vi "Process.vi"(8 "error in":errorcluster, 11 "SMO.SelfTerminating":refnum<class "SMO.SelfTerminating.lvclass">) -> (0 "error out":errorcluster, 3 "SMO.SelfTerminating out":refnum<class "SMO.SelfTerminating.lvclass">)   [LabVIEW 2013, in "SMO.SelfTerminating.lvclass"]
uses:
  SMO.SelfTerminating.lvclass
  SMO/Typedefs/Parent Call--Enum.ctl
  SMO/SMO.lvclass
panel:
  # "For instructions on how to use the JKI State Machine Objects, examples and video tutorials, visit:\nhttp://jki.net/state-machine-objects/\n\nJKI State Machine Objects™\nhttp://jki.net/state-machine-objects/\nCopyright (C) 2005-2015, JKI <info@jki.net>\nALL RIGHTS RESERVED"
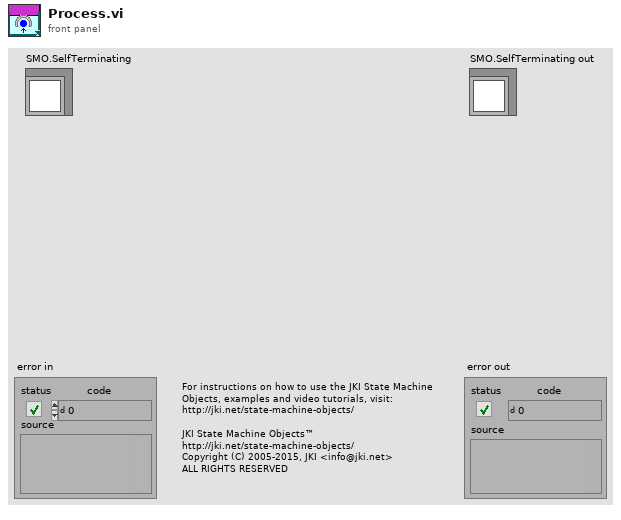
[diagram p1: front panel]
types:
  T1 = typedef "SMO.lvclass/Parent Call--Enum.ctl" = enum16{"Allows parent to run", "Does not request parent to run"}
  T2 = typedef "SMO.lvclass/Protected Events.ctl" = cluster{"StopProcesses":refnum<user-event>, "AbortProcesses":refnum<user-event>, "Config Changed":refnum<user-event>, "Dependency":refnum<user-event>}
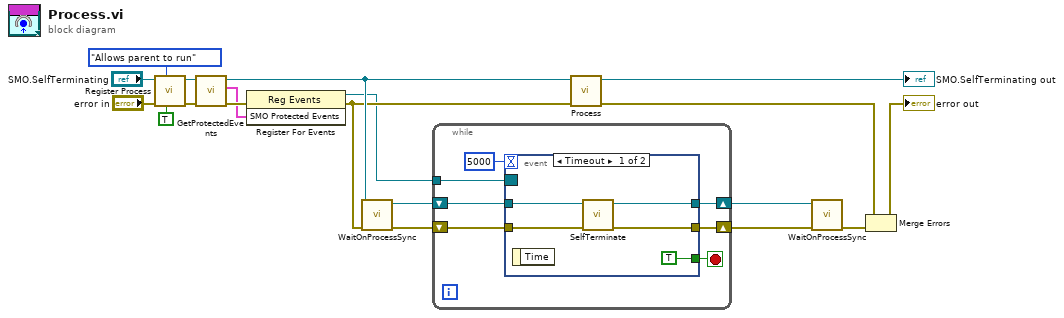
[diagram p0: block diagram]
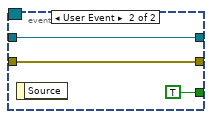
[diagram p2: hidden frame]
diagram:
  n1 = call "Register Process.vi"("Forces Self to Run (F)"=TRUE, "Parent Call"=Parent_Call--Enum."Allows parent to run", "error in (no error)"="error in", "SMO"="SMO.SelfTerminating") -> ("error out"=w9:errorcluster, "SMO out"=w11:refnum<class "SMO.SelfTerminating.lvclass">)  [unwired: 6 in]
  n2 = call "GetProtectedEvents.vi"("error in (no error)"=w9, "SMO"=w11) -> ("error out"=w8:errorcluster, "SMO Protected Events"=w6:T2, "SMO out"=w10:refnum<class "SMO.SelfTerminating.lvclass">)  [unwired: 7 in]
  n3 = register-events(error in=w8, w6) -> (reference out=w5:refnum<event-registration>, error out=w7:errorcluster)  [unwired: 1 in]
  n4 = call "WaitOnProcessSync.vi"("error in (no error)"=w7, "SMO"=w10) -> ("error out"=w3:errorcluster, "SMO out"=w4:refnum<class "SMO.SelfTerminating.lvclass">)  [unwired: 7 in, 1 out]
  n5 = while {
    tunnel: w5 -> [w25]
    shift-right: [w23] -> w2
    shift-left: w4 -> [w24]
    shift-right: [w21] -> w1
    shift-left: w3 -> [w22]
    stop <- w20 stop-if-true
    n6 = event shown="[0] Timeout" {
      selector: w25 -> [_ _]
      dyn-events: _ -> [_ _]
      timeout: 5000 -> [_ _]
      tunnel: w24 -> [w29 w34]
      tunnel: [w28 w34] -> w23
      tunnel: w22 -> [w30 w33]
      tunnel: [w27 w33] -> w21
      tunnel: [TRUE TRUE] -> w20
      event Timeout {
        n7 = event-data() -> ()  [unwired: 1 in, 1 out]
        n8 = call "SelfTerminate.vi"("error in (no error)"=w30, "SMO in"=w29) -> ("error out"=w27:errorcluster, "SMO out"=w28:refnum<class "SMO.SelfTerminating.lvclass">)  [unwired: 8 in]
      }
      event User Event {
        n9 = event-data() -> ()  [unwired: 1 in, 1 out]
      }
    }
  }
  n10 = call-parent "Process.vi"("error in"=w7, "SMO"=w10) -> ("error out"=w18:errorcluster, "SMO out"=→"SMO.SelfTerminating out":refnum<class "SMO.SelfTerminating.lvclass">)  [unwired: 8 in]
  n11 = call "WaitOnProcessSync.vi"("error in (no error)"=w1, "SMO"=w2) -> ("error out"=w12:errorcluster)  [unwired: 7 in, 2 out]
  n12 = Merge Errors(w18, w12) -> (→"error out":errorcluster)
